vi "Handle Listbox Shortcut Selection Event.vi"(8 "error in (no error)":errorcluster, 10 "Item Tag":string, 11 "dialog info in":T1={"steering frame ref"=refnum, "active wheel indexes"=[], "FP Refs"={"VI Refnum"=refnum, "Menu Ref"=refnum, "Sub Panel"=refnum, "picture"=refnum, "Steering Type"=refnum, "zoom in"=refnum, "zoom out"=refnum, "zoom extents"=refnum, "Wheels"=refnum, "Add Wheel"=refnum, "Remove Wheel"=refnum, "Copy Wheel"=refnum, "Angle Units"=refnum}, "subpanel info"={"subpanel VI refs"=[], "subpanel types"=[], "main to subpanel command events"=[]}, "picture dragging state"={"dragging"=FALSE, "wheel index"=-1, "dragging mode"=enum."translate", "wheel start position"={"x"=0.0, "y"=0.0, "theta"=0.0}, "relative mouse position"={"x"=0.0, "y"=0.0}, "relative mouse init angle (rad)"=0.0}, "picture size (pixels)"={"Width"=500, "Height"=500}, "picture grid"=bytes[0], "click zones group"={"click zones array"=[], "num click zones"=0}, "draw options"={"draw wheel states?"=FALSE, "highlight wheel index"=-1, "pixels per unit"=10.0, "draw forward velocity?"=FALSE, "velocity scale"=1.0}}) -> (0 "error out":errorcluster, 3 "dialog info out":T1={"steering frame ref"=refnum, "active wheel indexes"=[], "FP Refs"={"VI Refnum"=refnum, "Menu Ref"=refnum, "Sub Panel"=refnum, "picture"=refnum, "Steering Type"=refnum, "zoom in"=refnum, "zoom out"=refnum, "zoom extents"=refnum, "Wheels"=refnum, "Add Wheel"=refnum, "Remove Wheel"=refnum, "Copy Wheel"=refnum, "Angle Units"=refnum}, "subpanel info"={"subpanel VI refs"=[], "subpanel types"=[], "main to subpanel command events"=[]}, "picture dragging state"={"dragging"=FALSE, "wheel index"=-1, "dragging mode"=enum."translate", "wheel start position"={"x"=0.0, "y"=0.0, "theta"=0.0}, "relative mouse position"={"x"=0.0, "y"=0.0}, "relative mouse init angle (rad)"=0.0}, "picture size (pixels)"={"Width"=500, "Height"=500}, "picture grid"=bytes[0], "click zones group"={"click zones array"=[], "num click zones"=0}, "draw options"={"draw wheel states?"=FALSE, "highlight wheel index"=-1, "pixels per unit"=10.0, "draw forward velocity?"=FALSE, "velocity scale"=1.0}})   [LabVIEW 2017, in "NI_Robotics_Configure Steering Frame.lvlib"]
uses:
  <vilib>/robotics/Dialog/Configure Steering Frame/NI_Robotics_Configure Steering Frame.lvlib
  <vilib>/robotics/Dialog/Configure Steering Frame/Dialog Info.ctl
  <vilib>/robotics/Steering/Steering Frame/NI_Robotics_Steering Frame.lvclass
  <vilib>/robotics/Dialog/Configure Steering Frame/FP Refs.ctl
  <vilib>/robotics/Dialog/Configure Steering Frame/Subpanel Info.ctl
  <vilib>/robotics/Dialog/Configure Steering Frame/Main to Subpanel Command Event.ctl
  <vilib>/robotics/Dialog/Configure Steering Frame/Main to Subpanel Command.ctl
  <vilib>/robotics/Dialog/Configure Steering Frame/Dragging State.ctl
  <vilib>/robotics/Dialog/Configure Steering Frame/Dragging Mode.ctl
  <vilib>/Utility/miscctls.llb/LVBoundsTypeDef.ctl
  <vilib>/robotics/Dialog/Configure Steering Frame/Click Zone.ctl
  <vilib>/robotics/Utilities/Visualization/Steering Visualization/Steering Picture/Draw Steering Frame Options.ctl
  <vilib>/robotics/Utilities/Visualization/Steering Visualization/Steering Picture/NI_Robotics_Steering Picture.lvlib
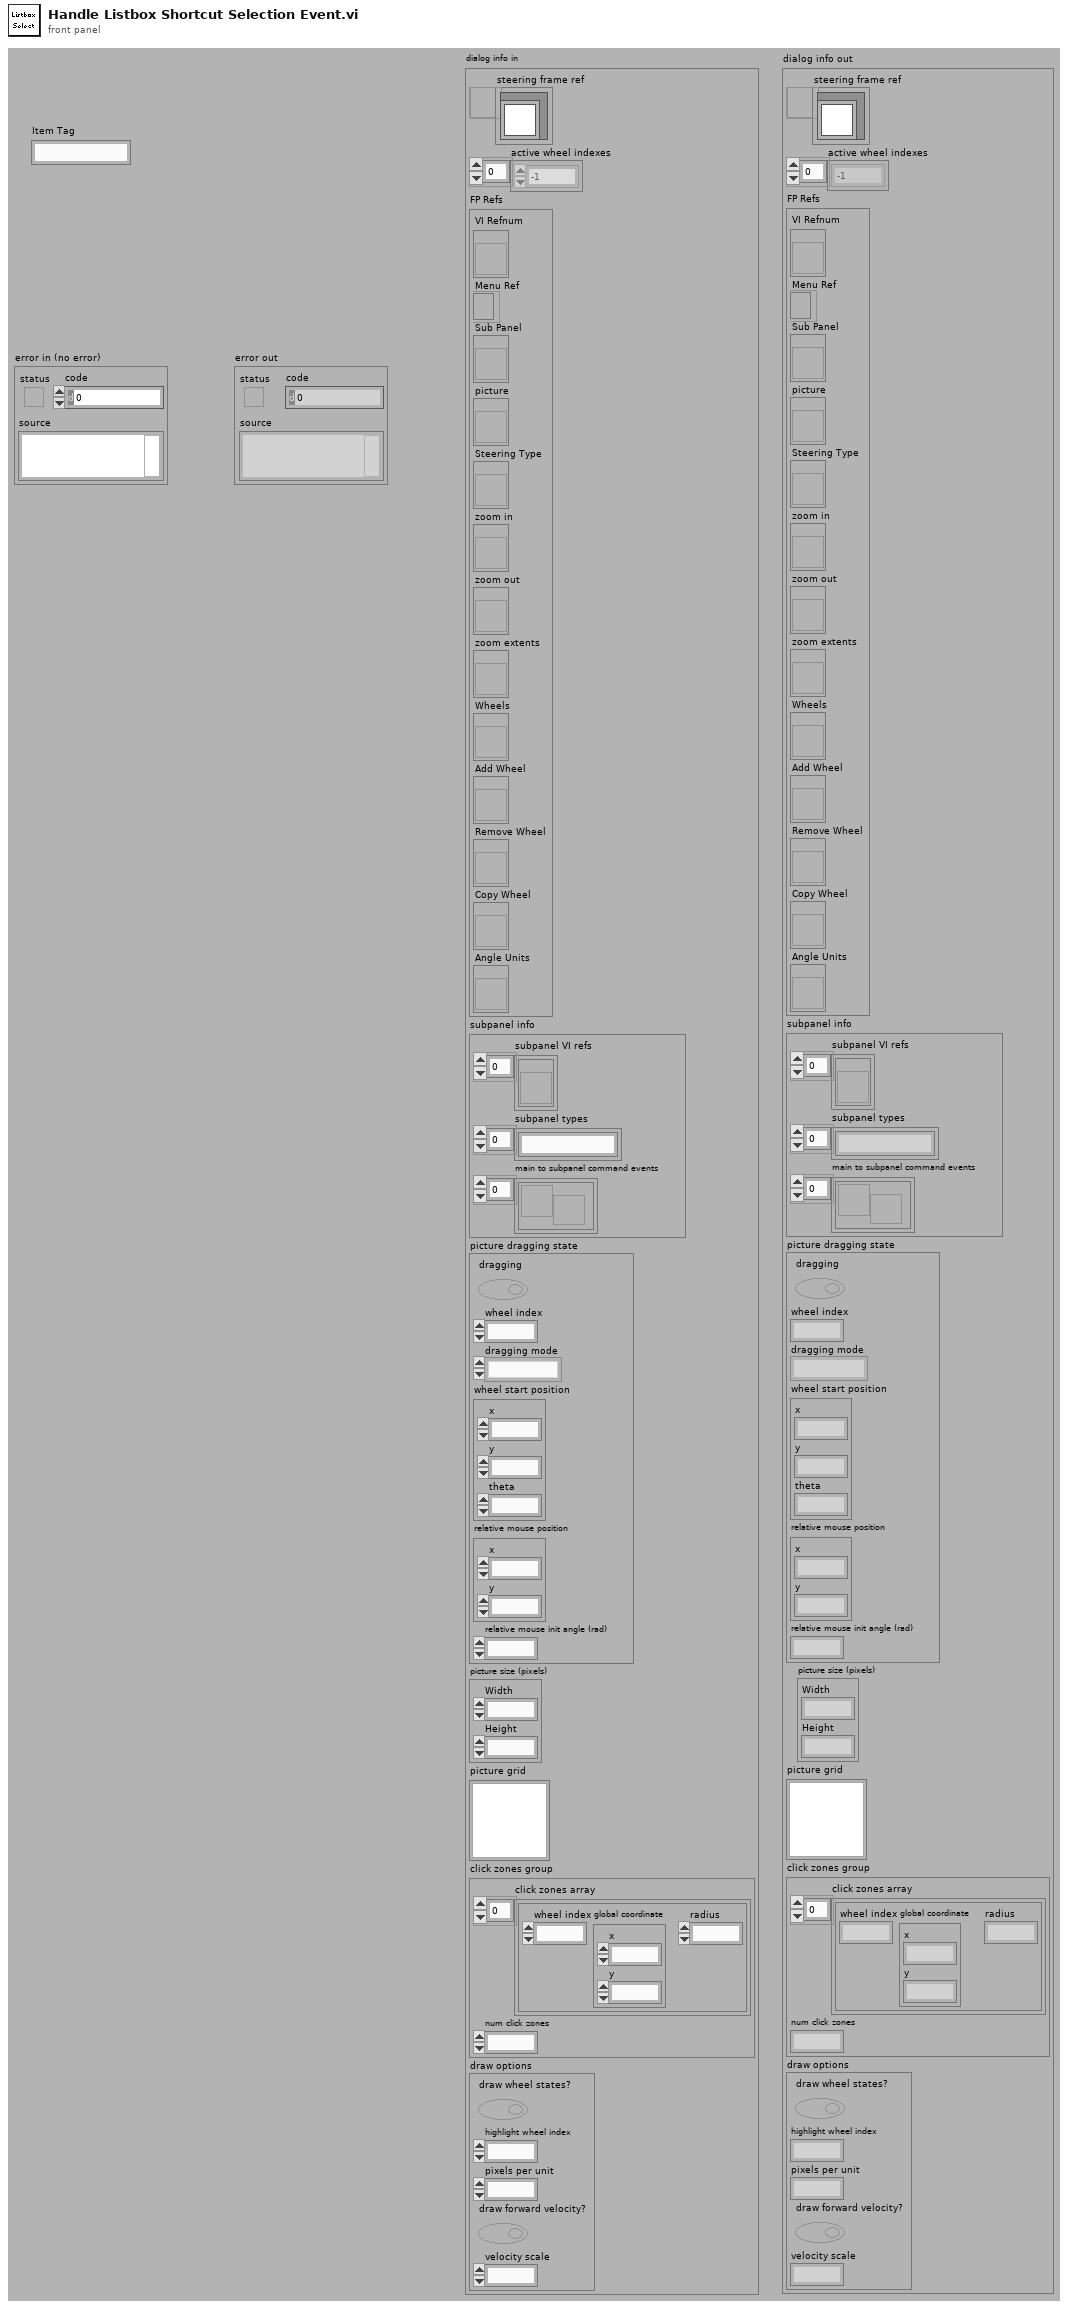
[diagram p1: front panel]
types:
  T1 = typedef "NI_Robotics_Configure Steering Frame.lvlib/Dialog Info.ctl" = cluster{"steering frame ref":refnum<data-value>, "active wheel indexes":i32[], "FP Refs":T2, "subpanel info":T3, "picture dragging state":T5, "picture size (pixels)":T7, "picture grid":picture, "click zones group":cluster{"click zones array":T8[], "num click zones":i32}, "draw options":T9}
  T2 = typedef "NI_Robotics_Configure Steering Frame.lvlib/FP Refs.ctl" = cluster{"VI Refnum":refnum<vi>, "Menu Ref":refnum<k9>, "Sub Panel":refnum<vi>, "picture":refnum<vi>, "Steering Type":refnum<vi>, "zoom in":refnum<vi>, "zoom out":refnum<vi>, "zoom extents":refnum<vi>, "Wheels":refnum<vi>, "Add Wheel":refnum<vi>, "Remove Wheel":refnum<vi>, "Copy Wheel":refnum<vi>, "Angle Units":refnum<vi>}
  T3 = typedef "NI_Robotics_Configure Steering Frame.lvlib/Subpanel Info.ctl" = cluster{"subpanel VI refs":refnum<vi>[], "subpanel types":string[], "main to subpanel command events":T4[]}
  T4 = typedef "NI_Robotics_Configure Steering Frame.lvlib/Main to Subpanel Command Event.ctl" = refnum<user-event>
  T5 = typedef "NI_Robotics_Configure Steering Frame.lvlib/Dragging State.ctl" = cluster{"dragging":bool, "wheel index":i32, "dragging mode":T6, "wheel start position":cluster{"x":dbl, "y":dbl, "theta":dbl}, "relative mouse position":cluster{"x":dbl, "y":dbl}, "relative mouse init angle (rad)":dbl}
  T6 = typedef "NI_Robotics_Configure Steering Frame.lvlib/Dragging Mode.ctl" = enum16{"translate", "rotate"}
  T7 = typedef "LVBoundsTypeDef.ctl" = cluster{"Width":u32, "Height":u32}
  T8 = typedef "NI_Robotics_Configure Steering Frame.lvlib/Click Zone.ctl" = cluster{"wheel index":i32, "global coordinate":cluster{"x":dbl, "y":dbl}, "radius":dbl}
  T9 = typedef "NI_Robotics_Steering Picture.lvlib/Draw Steering Frame Options.ctl" = cluster{"draw wheel states?":bool, "highlight wheel index":i32, "pixels per unit":dbl, "draw forward velocity?":bool, "velocity scale":dbl}
  T10 = enum16{"open", "replace", "create", "open or create", "replace or create", "replace or create with confirmation"}
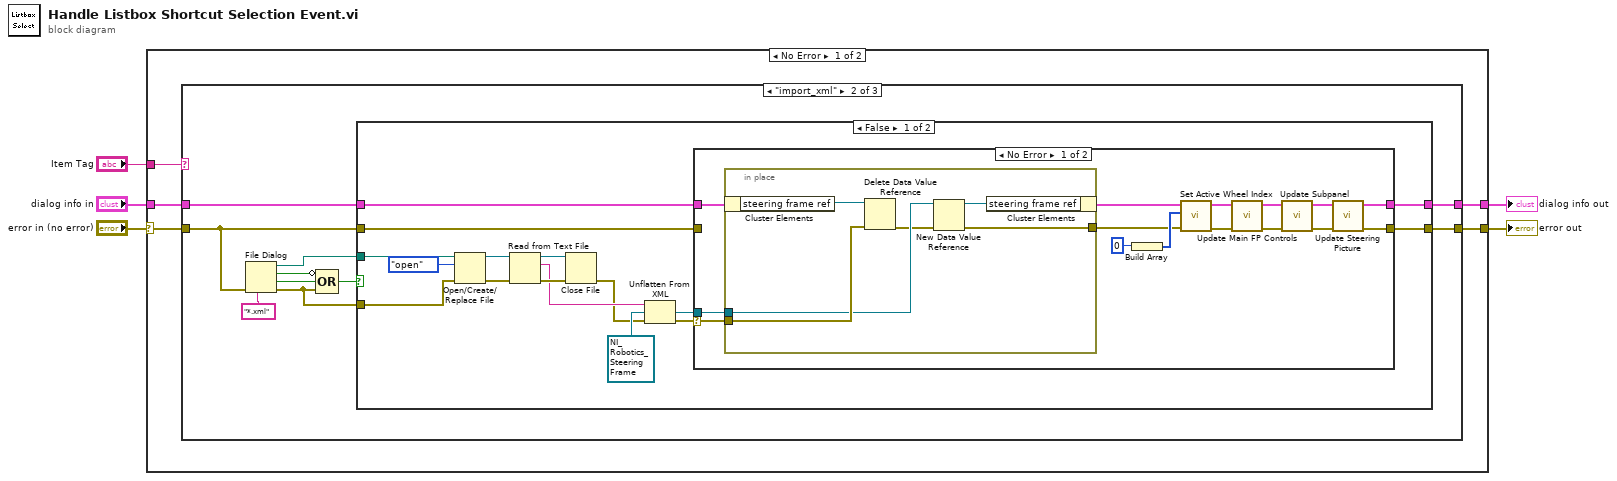
[diagram p0: block diagram]
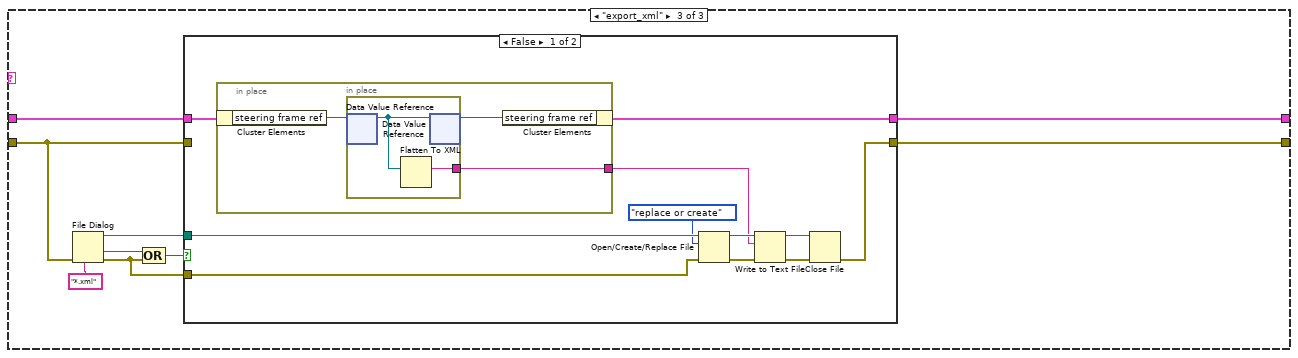
[diagram p5: hidden frame]
diagram:
  n1 = case shown="No Error" "error in (no error)" {
    selector: "error in (no error)" -> [w8 w91]
    tunnel: "dialog info in" -> [w9 w92]
    tunnel: [w7 w92] -> w3
    tunnel: [w6 w91] -> w2
    tunnel: "Item Tag" -> [w10 _]
    frame No Error {
      n2 = case shown="\"import_xml\"" w10 {
        tunnel: w9 -> [w12 w18 w69]
        tunnel: w8 -> [w11 w16 w67]
        tunnel: [w12 w17 w68] -> w7
        tunnel: [w11 w15 w66] -> w6
        frame Default {
        }
        frame "import_xml" {
          n3 = File Dialog(6:"*.xml" ("pattern (all files)"), 8:w16) -> (0:w14:errorcluster, 1:w21:bool, 2:w20:bool, 3:w13:path)  [unwired: 5 in]
          n4 = Compound Arithmetic op=OR(invert w20, w21, w14) -> (w19:bool)
          n5 = case shown="False" w19 {
            tunnel: w18 -> [w27 w62]
            tunnel: [w26 w62] -> w17
            tunnel: w16 -> [w23 w63]
            tunnel: [w24 w63] -> w15
            tunnel: w14 -> [w36 _]
            tunnel: w13 -> [w38 _]
            frame False {
              n6 = Open/Create/Replace File(file path (use dialog)=w38, error in=w36, operation (0:open)=T10."open") -> (refnum out=w35:refnum<file>, error out=w34:errorcluster)  [unwired: 3 in, 1 out]
              n7 = Read from Text File(file (use dialog)=w35, error in=w34) -> (refnum out=w33:refnum<file>, text=w31:string, error out=w32:errorcluster)  [unwired: 2 in, 1 out]
              n8 = Close File(refnum=w33, error in=w32) -> (error out=w25:errorcluster)  [unwired: 1 out]
              n9 = Unflatten From XML(xml string=w31, type=refnum<class "NI_Robotics_Steering Frame.lvclass"> refnum ("NI_Robotics_Steering Frame.lvclass"), error in (no error)=w25) -> (value=w28:refnum<class "NI_Robotics_Steering Frame.lvclass">, error out=w29:errorcluster)
              n10 = case shown="No Error" w29 {
                selector: w29 -> [w51 _]
                tunnel: w28 -> [w52 _]
                tunnel: w27 -> [w53 w61]
                tunnel: [w41 w61] -> w26
                tunnel: [w39 w60] -> w24
                tunnel: w23 -> [_ w60]
                frame No Error {
                  n11 = in-place {
                    in-place-border: w52 -> [w56]
                    in-place-border: w51 -> [w58]
                    in-place-border: [w54] -> w47
                    n12 = in-place-cluster #1(w53) -> ("steering frame ref"=w59:refnum<data-value>)
                    n13 = Delete Data Value Reference(data value reference=w59, error in=w58) -> (error out=w55:errorcluster)  [unwired: 1 out]
                    n14 = New Data Value Reference(data value=w56, error in=w55) -> (data value reference=w57:refnum<data-value>, error out=w54:errorcluster)
                    n15 = in-place-cluster #1("steering frame ref"=w57) -> (w48:T1)
                  }
                  n16 = Build Array(0) -> (w50:i32[])
                  n17 = call <vilib>:"Set Active Wheel Index.vi"("error in (no error)"=w47, "active wheel indexes"=w50, "dialog info in"=w48) -> ("error out"=w40:errorcluster, "dialog info out"=w42:T1)  [unwired: 7 in]
                  n18 = call <vilib>:"Update Main FP Controls.vi"("error in (no error)"=w40, "dialog info in"=w42) -> ("error out"=w46:errorcluster, "dialog info out"=w45:T1)  [unwired: 8 in]
                  n19 = call <vilib>:"Update Subpanel.vi"("error in (no error)"=w46, "dialog info in"=w45) -> ("error out"=w44:errorcluster, "dialog info out"=w43:T1)  [unwired: 8 in]
                  n20 = call <vilib>:"Update Steering Picture.vi"("error in (no error)"=w44, "dialog info in"=w43) -> ("error out"=w39:errorcluster, "dialog info out"=w41:T1)  [unwired: 8 in]
                }
                frame Error {
                }
              }
            }
            frame True {
            }
          }
        }
        frame "export_xml" {
          n21 = File Dialog(6:"*.xml" ("pattern (all files)"), 8:w67) -> (0:w65:errorcluster, 1:w71:bool, 3:w64:path)  [unwired: 5 in, 1 out]
          n22 = Compound Arithmetic op=OR(w71, w65) -> (w70:bool)
          n23 = case shown="False" w70 {
            tunnel: w69 -> [w80 w89]
            tunnel: [w79 w89] -> w68
            tunnel: w67 -> [_ w90]
            tunnel: [w73 w90] -> w66
            tunnel: w65 -> [w81 _]
            tunnel: w64 -> [w83 _]
            frame False {
              n24 = in-place {
                in-place-border: [w84] -> w74
                n25 = in-place-cluster #2(w80) -> ("steering frame ref"=w86:refnum<data-value>)
                n26 = in-place {
                  in-place-border: [w87] -> w84
                  n27 = in-place-dvr #3(w86) -> (w88:refnum<class "NI_Robotics_Steering Frame.lvclass">)  [unwired: 1 out]
                  n28 = Flatten To XML(anything=w88) -> (xml string=w87:string)
                  n29 = in-place-dvr #3(w88) -> (w85:refnum<data-value>)  [unwired: 1 out]
                }
                n30 = in-place-cluster #2("steering frame ref"=w85) -> (w79:T1)
              }
              n31 = Open/Create/Replace File(file path (use dialog)=w83, error in=w81, operation (0:open)=T10."replace or create") -> (refnum out=w78:refnum<file>, error out=w77:errorcluster)  [unwired: 3 in, 1 out]
              n32 = Write to Text File(file (use dialog)=w78, text=w74, error in=w77) -> (refnum out=w76:refnum<file>, error out=w75:errorcluster)  [unwired: 1 in, 1 out]
              n33 = Close File(refnum=w76, error in=w75) -> (error out=w73:errorcluster)  [unwired: 1 out]
            }
            frame True {
            }
          }
        }
      }
    }
    frame Error {
    }
  }
  "error out" <- w2
  "dialog info out" <- w3
